vi "运维调试界面.vi"() -> ()   [LabVIEW 2016, in "质控单元V2.lvlib"]
uses:
  <vilib>/Utility/miscctls.llb/LVPointTypeDef.ctl
panel:
  in  "周期设置":bool
  in  "集成干预测试":bool
  in  "平行样测试":bool
  in  "水样测试":bool
  in  "数值":u8
  in  "向前寻道按钮":bool
  in  "向后寻道按钮":bool
  out "质控状态 4":T1
  out "质控状态 3":T1
  out "质控状态 2":T1
  out "质控状态":T1
  out "权限等级":string
  in  "布尔":bool
  out "模块版本号":string
  in  "停止":bool
  in  "参数设置":bool
  in  "连接设置":bool
  in  "调试界面":bool
  in  "加标回收":bool
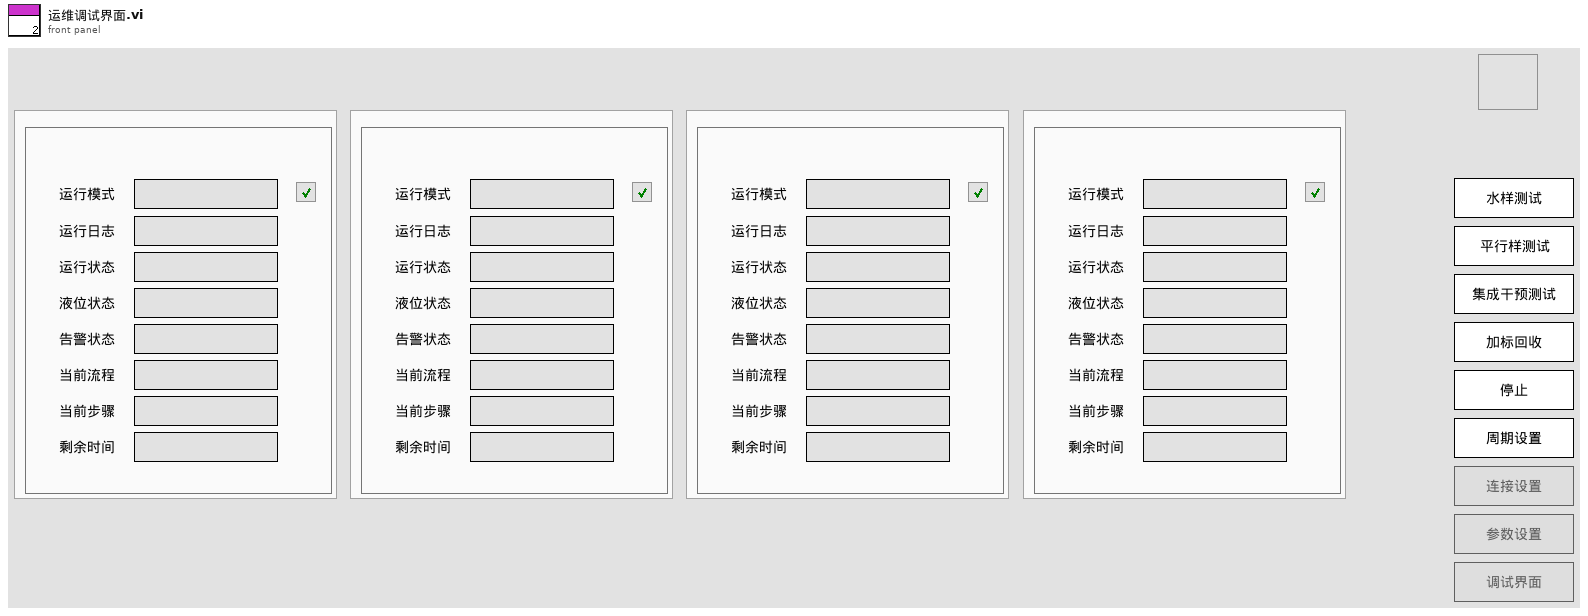
[diagram p1: front panel]
types:
  T1 = typedef "质控单元V2.lvlib/质控状态.ctl" = cluster{"模块名称":string, "通讯状态":bool, "运行模式":string, "运行日志":string, "运行状态":string, "液位状态":string, "告警状态":string, "当前流程":string, "当前步骤":string, "剩余时间":string}
  T2 = typedef "质控单元V2.lvlib/数据流类型.ctl" = cluster{"cmd":enum16{"start", "stop"}, "data":variant}
  T3 = typedef "LVPointTypeDef.ctl" = cluster{"Horizontal":i16, "Vertical":i16}
  T4 = typedef "质控单元V2.lvlib/质控仪器状态显示.ctl" = cluster{"运行模式":string, "运行状态":string, "液位状态":string, "告警状态":string, "当前流程":string, "当前步骤":string, "剩余时间":string}
  T5 = cluster{"氨氮":bool, "总磷":bool, "总氮":bool, "CODMn":bool, "CODCr":bool, "氨氮总磷":bool, "总磷总氮":bool}
  T6 = typedef "质控单元V2.lvlib/质控slave id.ctl" = enum16{"null", "氨氮", "总磷", "总氮", "CODMn", "CODCr"}
  T7 = typedef "质控单元V2.lvlib/测试流程.ctl" = enum16{"加标回收（启动采配水）", "加标回收（不启动采配水）", "水样测试（启动采配水）", "水样测试（不启动采配水）", "平行样测试（启动采配水）", "平行样测试（不启动采配水）", "集成干预测试"}
  T8 = cluster{"启用参数选择":cluster{"氨氮启用":bool, "总磷启用":bool, "总氮启用":bool, "CODMn启用":bool, "CODCr启用":bool}, "流程":T7}
  T9 = cluster{"氨氮启用":bool, "总磷启用":bool, "总氮启用":bool, "CODMn启用":bool, "CODCr启用":bool}
  T10 = enum8{"Enabled", "Disabled", "Disabled and Grayed Out"}
  T11 = cluster{"Major":u16, "Minor":u16, "Fix":u16, "Build":u16}
  T12 = cluster{"氨氮":bool, "总磷":bool, "总氮":bool, "CODMn":bool, "CODCr":bool}
  T13 = cluster{"氨氮":bool, "总磷":bool, "总氮":bool, "CODMn":bool, "CODCr":bool, bool, bool}
  T14 = typedef "ZKTimingControl.lvlib/TimingControl.lvclass/国标控制命令.ctl" = enum16{"加标回收（启动采配水）", "加标回收（不启动采配水）", "水样测试（启动采配水）", "水样测试（不启动采配水）", "平行样测试（启动采配水）", "平行样测试（不启动采配水）", "集成干预测试"}
  T15 = typedef "ZKTimingControl.lvlib/TimingControl.lvclass/测量参数.ctl" = cluster{"氨氮":bool, "总磷":bool, "总氮":bool, "CODMn":bool, "CODCr":bool, "氟化物":bool, "挥发酚":bool}
  T16 = enum32{"Bad", "Idle", "Run top level", "Running"}
  T17 = cluster{"启动参数":cluster{"氨氮启用":bool, "总磷启用":bool, "总氮启用":bool, "CODMn启用":bool, "CODCr启用":bool}, "流程参数":T7}
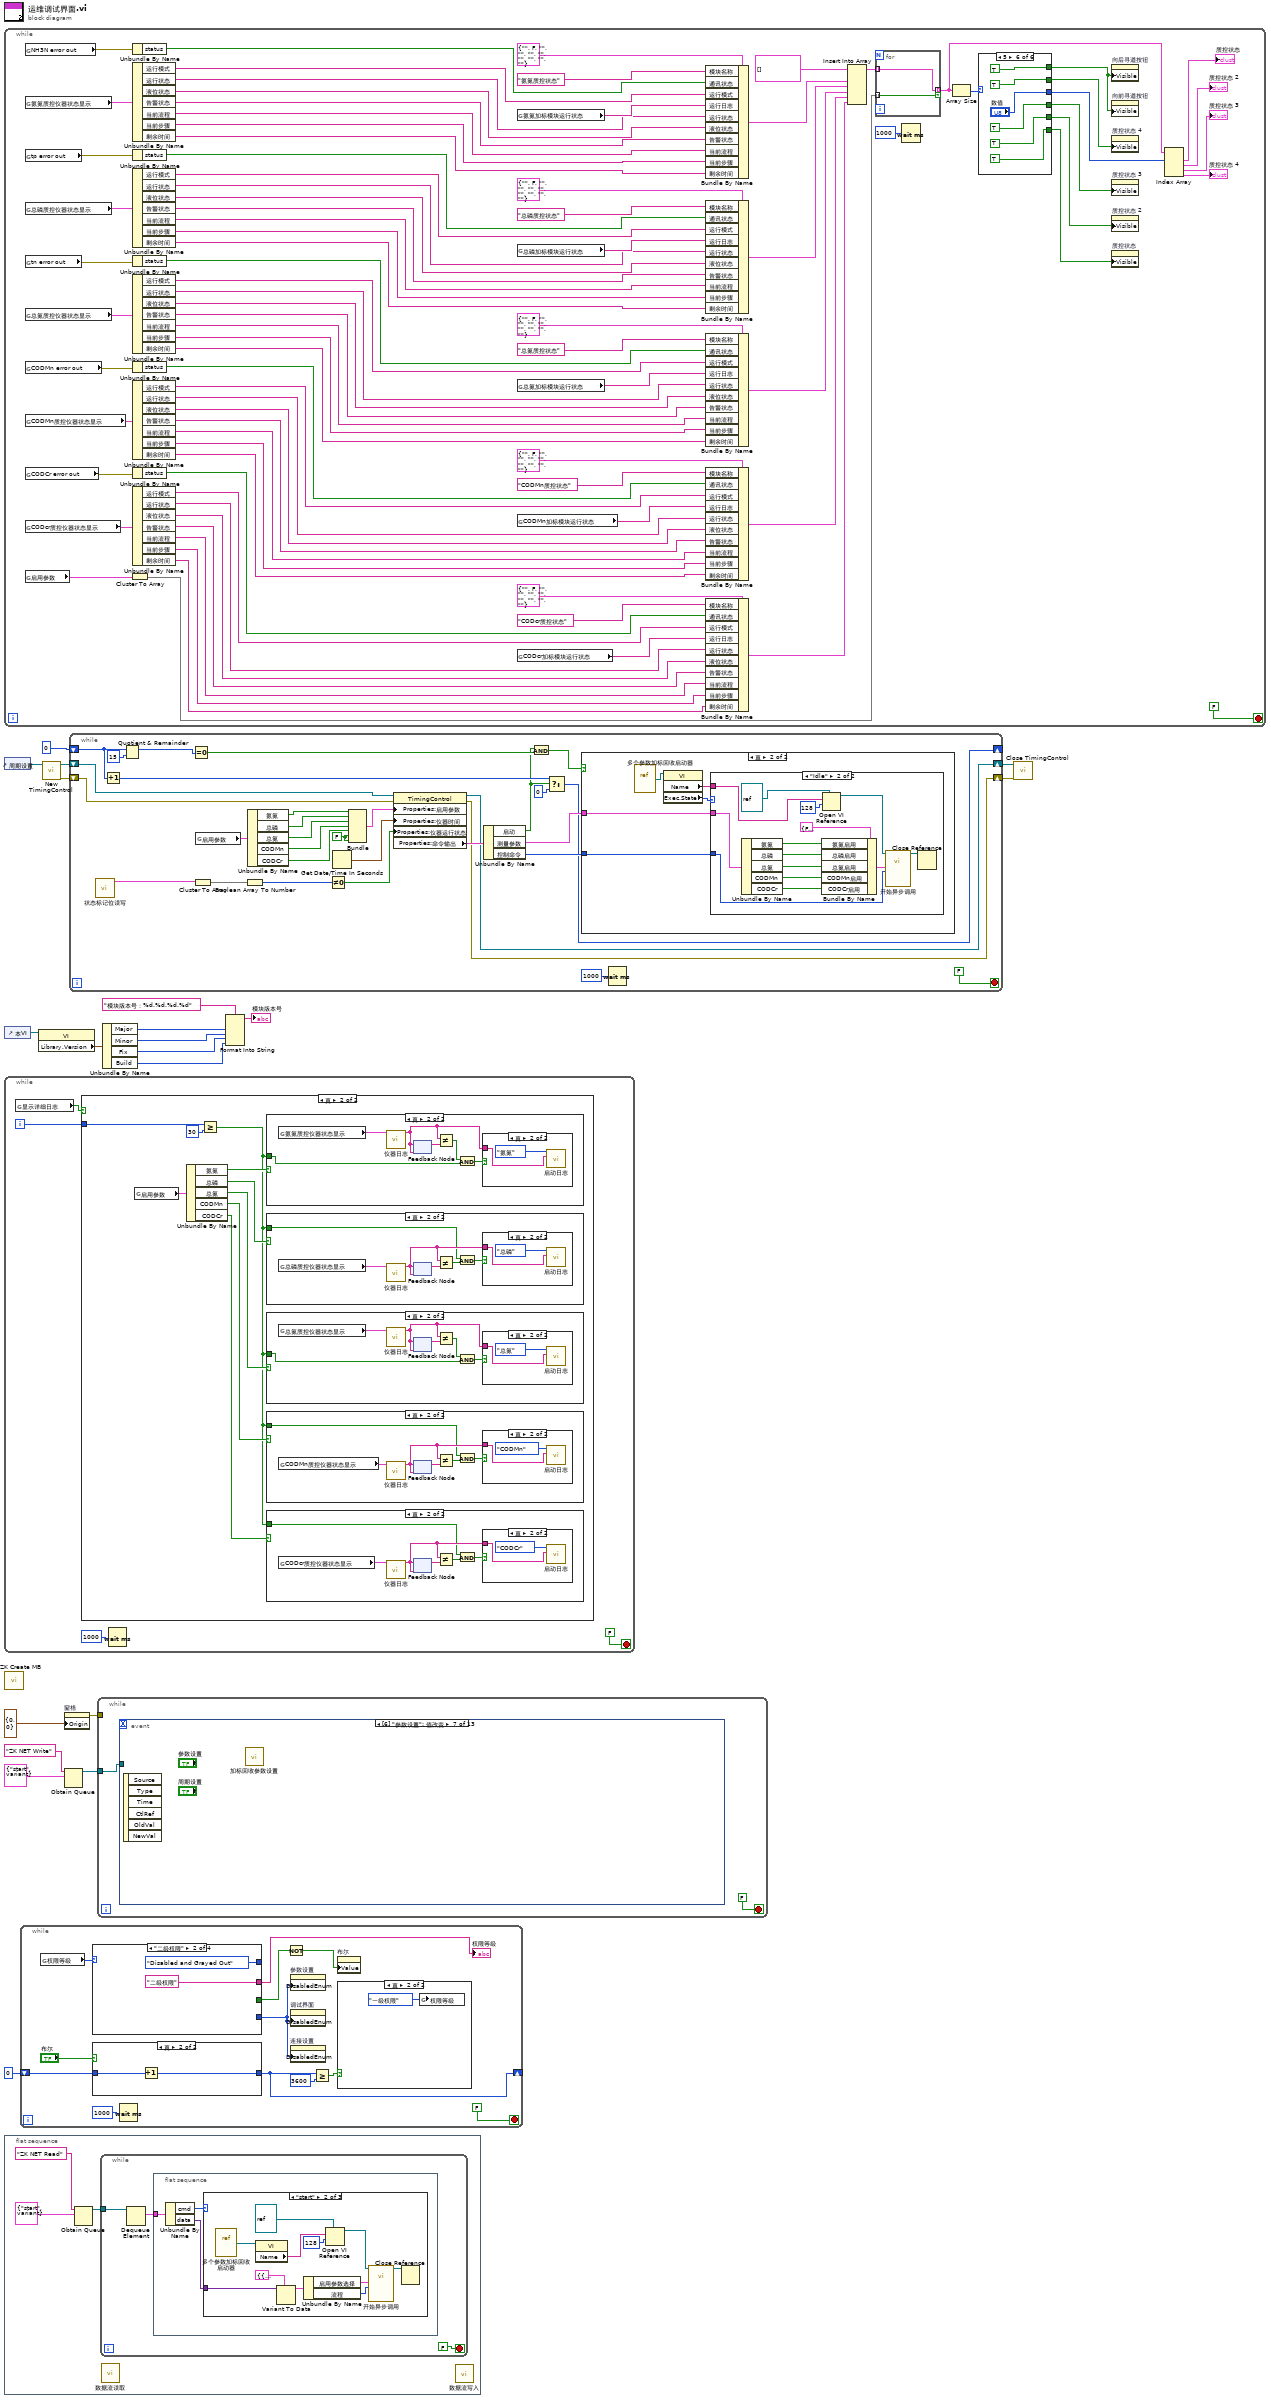
[diagram p0: block diagram]
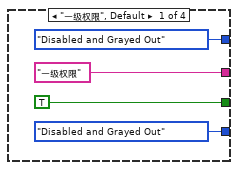
[diagram p13: hidden frame]
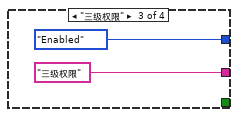
[diagram p14: hidden frame]
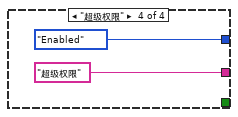
[diagram p15: hidden frame]
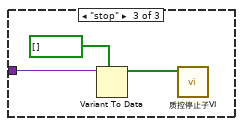
[diagram p19: hidden frame]
diagram:
  n1 = while {
    stop <- FALSE stop-if-true
    n2 = global read "ZK非断电保存全局变量.vi" "NH3N error out"() -> (w105:errorcluster)
    n3 = global read "ZK非断电保存全局变量.vi" "氨氮质控仪器状态显示"() -> (w104:T4)
    n4 = global read "ZK非断电保存全局变量.vi" "tp error out"() -> (w100:errorcluster)
    n5 = global read "ZK非断电保存全局变量.vi" "总磷质控仪器状态显示"() -> (w103:T4)
    n6 = global read "ZK非断电保存全局变量.vi" "tn error out"() -> (w99:errorcluster)
    n7 = global read "ZK非断电保存全局变量.vi" "总氮质控仪器状态显示"() -> (w102:T4)
    n8 = global read "ZK非断电保存全局变量.vi" "CODMn error out"() -> (w106:errorcluster)
    n9 = global read "ZK非断电保存全局变量.vi" "CODMn质控仪器状态显示"() -> (w101:T4)
    n10 = global read "ZK非断电保存全局变量.vi" "CODCr error out"() -> (w37:errorcluster)
    n11 = global read "ZK非断电保存全局变量.vi" "CODcr质控仪器状态显示"() -> (w38:T4)
    n12 = global read "ZK断电保存全局变量.vi" "启用参数"() -> (w34:T5)
    n13 = Cluster To Array(cluster=w34) -> (array=w33:bool[])
    n14 = Unbundle By Name(w105) -> ("status"=w97:bool)
    n15 = Unbundle By Name(w104) -> ("运行模式"=w95:string, "运行状态"=w93:string, "液位状态"=w92:string, "告警状态"=w91:string, "当前流程"=w90:string, "当前步骤"=w89:string, "剩余时间"=w88:string)
    n16 = Unbundle By Name(w100) -> ("status"=w77:bool)
    n17 = Unbundle By Name(w103) -> ("运行模式"=w85:string, "运行状态"=w84:string, "液位状态"=w83:string, "告警状态"=w82:string, "当前流程"=w81:string, "当前步骤"=w80:string, "剩余时间"=w79:string)
    n18 = Unbundle By Name(w99) -> ("status"=w61:bool)
    n19 = Unbundle By Name(w102) -> ("运行模式"=w63:string, "运行状态"=w60:string, "液位状态"=w59:string, "告警状态"=w58:string, "当前流程"=w57:string, "当前步骤"=w56:string, "剩余时间"=w55:string)
    n20 = Unbundle By Name(w106) -> ("status"=w74:bool)
    n21 = Unbundle By Name(w101) -> ("运行模式"=w72:string, "运行状态"=w71:string, "液位状态"=w70:string, "告警状态"=w69:string, "当前流程"=w68:string, "当前步骤"=w67:string, "剩余时间"=w66:string)
    n22 = Unbundle By Name(w37) -> ("status"=w41:bool)
    n23 = Unbundle By Name(w38) -> ("运行模式"=w43:string, "运行状态"=w44:string, "液位状态"=w45:string, "告警状态"=w46:string, "当前流程"=w47:string, "当前步骤"=w48:string, "剩余时间"=w49:string)
    n24 = global read "ZK非断电保存全局变量.vi" "氨氮加标模块运行状态"() -> (w94:string)
    n25 = global read "ZK非断电保存全局变量.vi" "总磷加标模块运行状态"() -> (w86:string)
    n26 = global read "ZK非断电保存全局变量.vi" "总氮加标模块运行状态"() -> (w62:string)
    n27 = global read "ZK非断电保存全局变量.vi" "CODMn加标模块运行状态"() -> (w73:string)
    n28 = global read "ZK非断电保存全局变量.vi" "CODcr加标模块运行状态"() -> (w42:string)
    n29 = Bundle By Name(cluster=T1 {"模块名称"="", "通讯状态"=FALSE, "运行模式"="", "运行日志"="", "运行状态"="", "液位状态"="", "告警状态"="", "当前流程"="", "当前步骤"="", "剩余时间"=""} ("质控状态"), "模块名称"="氨氮质控状态", "通讯状态"=w97, "运行模式"=w95, "运行日志"=w94, "运行状态"=w93, "液位状态"=w92, "告警状态"=w91, "当前流程"=w90, "当前步骤"=w89, "剩余时间"=w88) -> (w54:T1)
    n30 = Bundle By Name(cluster=T1 {"模块名称"="", "通讯状态"=FALSE, "运行模式"="", "运行日志"="", "运行状态"="", "液位状态"="", "告警状态"="", "当前流程"="", "当前步骤"="", "剩余时间"=""} ("质控状态"), "模块名称"="总磷质控状态", "通讯状态"=w77, "运行模式"=w85, "运行日志"=w86, "运行状态"=w84, "液位状态"=w83, "告警状态"=w82, "当前流程"=w81, "当前步骤"=w80, "剩余时间"=w79) -> (w52:T1)
    n31 = Bundle By Name(cluster=T1 {"模块名称"="", "通讯状态"=FALSE, "运行模式"="", "运行日志"="", "运行状态"="", "液位状态"="", "告警状态"="", "当前流程"="", "当前步骤"="", "剩余时间"=""} ("质控状态"), "模块名称"="总氮质控状态", "通讯状态"=w61, "运行模式"=w63, "运行日志"=w62, "运行状态"=w60, "液位状态"=w59, "告警状态"=w58, "当前流程"=w57, "当前步骤"=w56, "剩余时间"=w55) -> (w51:T1)
    n32 = Bundle By Name(cluster=T1 {"模块名称"="", "通讯状态"=FALSE, "运行模式"="", "运行日志"="", "运行状态"="", "液位状态"="", "告警状态"="", "当前流程"="", "当前步骤"="", "剩余时间"=""} ("质控状态"), "模块名称"="CODMn质控状态", "通讯状态"=w74, "运行模式"=w72, "运行日志"=w73, "运行状态"=w71, "液位状态"=w70, "告警状态"=w69, "当前流程"=w68, "当前步骤"=w67, "剩余时间"=w66) -> (w50:T1)
    n33 = Bundle By Name(cluster=T1 {"模块名称"="", "通讯状态"=FALSE, "运行模式"="", "运行日志"="", "运行状态"="", "液位状态"="", "告警状态"="", "当前流程"="", "当前步骤"="", "剩余时间"=""} ("质控状态"), "模块名称"="CODcr质控状态", "通讯状态"=w41, "运行模式"=w43, "运行日志"=w42, "运行状态"=w44, "液位状态"=w45, "告警状态"=w46, "当前流程"=w47, "当前步骤"=w48, "剩余时间"=w49) -> (w36:T1)
    n34 = Insert Into Array(array=T1[] [] ("数组"), new element #1=w54, new element #2=w52, new element #3=w51, new element #4=w50, new element #5=w36) -> (w35:T1[])  [unwired: 1 in]
    n35 = for {
      tunnel: w35 -> [w130] mode=indexing
      tunnel: w33 -> [w129] mode=indexing
      tunnel: [w130] -> w28 mode=indexing if=w129
    }
    n36 = Wait (ms)(milliseconds to wait=u32 1000 ("等待时间（毫秒）")) -> ()  [unwired: 1 out]
    n37 = Array Size(array=w28) -> (size(s)=w27:i32)
    n38 = case shown="5" w27 {
      tunnel: [FALSE TRUE TRUE TRUE TRUE TRUE] -> w26
      tunnel: [FALSE _ TRUE TRUE TRUE TRUE] -> w25
      tunnel: [FALSE _ _ TRUE TRUE TRUE] -> w24
      tunnel: [FALSE _ _ _ TRUE TRUE] -> w23
      tunnel: [_ _ _ _ _ TRUE] -> w22
      tunnel: [_ _ _ _ _ "数值"] -> w21
      frame 0, Default {
      }
      frame 1 {
      }
      frame 2 {
      }
      frame 3 {
      }
      frame 4 {
      }
      frame 5 {
      }
    }
    n39 = property on="向后寻道按钮" class="Bool"("Visible"=w22) -> ()  [unwired: 2 in, 2 out]
    n40 = property on="向前寻道按钮" class="Bool"("Visible"=w22) -> ()  [unwired: 2 in, 2 out]
    n41 = property on="质控状态 4" class="Clust (严格)"("Visible"=w23) -> ()  [unwired: 2 in, 2 out]
    n42 = property on="质控状态 3" class="Clust (严格)"("Visible"=w24) -> ()  [unwired: 2 in, 2 out]
    n43 = property on="质控状态 2" class="Clust (严格)"("Visible"=w25) -> ()  [unwired: 2 in, 2 out]
    n44 = property on="质控状态" class="Clust (严格)"("Visible"=w26) -> ()  [unwired: 2 in, 2 out]
    n45 = Index Array(array=w28, index #1=w21) -> (element #1=→"质控状态":T1, element #2=→"质控状态 2":T1, element #3=→"质控状态 3":T1, element #4=→"质控状态 4":T1)  [unwired: 3 in]
  }
  n46 = control-ref of="周期设置"() -> (w1:refnum<vi>)
  n47 = control-ref of="本VI"() -> (w18:refnum<vi>)
  n48 = while {
    i -> [w132]
    stop <- FALSE stop-if-true
    n49 = global read "ZK断电保存全局变量.vi" "显示详细日志"() -> (w131:bool)
    n50 = case shown="真" w131 {
      tunnel: w132 -> [_ w137]
      frame False {
      }
      frame True {
        n51 = global read "ZK断电保存全局变量.vi" "启用参数"() -> (w143:T5)
        n52 = Unbundle By Name(w143) -> ("氨氮"=w142:bool, "总磷"=w141:bool, "总氮"=w140:bool, "CODMn"=w139:bool, "CODCr"=w138:bool)
        n53 = Greater Or Equal?(x=w137, y=30) -> (x >= y?=w135:bool)
        n54 = case shown="真" w142 {
          tunnel: w135 -> [_ w176]
          frame False {
          }
          frame True {
            n55 = global read "ZK非断电保存全局变量.vi" "氨氮质控仪器状态显示"() -> (w181:T4)
            n56 = call "仪器日志.vi"("质控仪器状态显示"=w181) -> ("仪器日志"=w179:string)  [unwired: 10 in]
            n57 = feedback-in #1(w179) -> ()
            n58 = feedback #1(w179) -> (w180:string)
            n59 = Not Equal?(x=w179, y=w180) -> (x != y?=w178:bool)
            n60 = And(x=w178, y=w176) -> (x .and. y?=w177:bool)
            n61 = case shown="真" w177 {
              tunnel: w179 -> [_ w182]
              frame False {
              }
              frame True {
                n62 = call "启动日志.vi"("日志信息"=w182, "Slave ID"=质控slave_id."氨氮") -> ()  [unwired: 9 in, 1 out]
              }
            }
          }
        }
        n63 = case shown="真" w141 {
          tunnel: w135 -> [_ w168]
          frame False {
          }
          frame True {
            n64 = global read "ZK非断电保存全局变量.vi" "总磷质控仪器状态显示"() -> (w170:T4)
            n65 = call "仪器日志.vi"("质控仪器状态显示"=w170) -> ("仪器日志"=w172:string)  [unwired: 10 in]
            n66 = feedback #2(w172) -> (w173:string)
            n67 = feedback-in #2(w172) -> ()
            n68 = Not Equal?(x=w172, y=w173) -> (x != y?=w171:bool)
            n69 = And(x=w168, y=w171) -> (x .and. y?=w169:bool)
            n70 = case shown="真" w169 {
              tunnel: w172 -> [_ w174]
              frame False {
              }
              frame True {
                n71 = call "启动日志.vi"("日志信息"=w174, "Slave ID"=质控slave_id."总磷") -> ()  [unwired: 9 in, 1 out]
              }
            }
          }
        }
        n72 = case shown="真" w140 {
          tunnel: w135 -> [_ w160]
          frame False {
          }
          frame True {
            n73 = global read "ZK非断电保存全局变量.vi" "总氮质控仪器状态显示"() -> (w162:T4)
            n74 = call "仪器日志.vi"("质控仪器状态显示"=w162) -> ("仪器日志"=w164:string)  [unwired: 10 in]
            n75 = feedback #3(w164) -> (w165:string)
            n76 = feedback-in #3(w164) -> ()
            n77 = Not Equal?(x=w164, y=w165) -> (x != y?=w163:bool)
            n78 = And(x=w163, y=w160) -> (x .and. y?=w161:bool)
            n79 = case shown="真" w161 {
              tunnel: w164 -> [_ w166]
              frame False {
              }
              frame True {
                n80 = call "启动日志.vi"("日志信息"=w166, "Slave ID"=质控slave_id."总氮") -> ()  [unwired: 9 in, 1 out]
              }
            }
          }
        }
        n81 = case shown="真" w139 {
          tunnel: w135 -> [_ w152]
          frame False {
          }
          frame True {
            n82 = global read "ZK非断电保存全局变量.vi" "CODMn质控仪器状态显示"() -> (w154:T4)
            n83 = call "仪器日志.vi"("质控仪器状态显示"=w154) -> ("仪器日志"=w156:string)  [unwired: 10 in]
            n84 = feedback #4(w156) -> (w157:string)
            n85 = feedback-in #4(w156) -> ()
            n86 = Not Equal?(x=w156, y=w157) -> (x != y?=w155:bool)
            n87 = And(x=w152, y=w155) -> (x .and. y?=w153:bool)
            n88 = case shown="真" w153 {
              tunnel: w156 -> [_ w158]
              frame False {
              }
              frame True {
                n89 = call "启动日志.vi"("日志信息"=w158, "Slave ID"=质控slave_id."CODMn") -> ()  [unwired: 9 in, 1 out]
              }
            }
          }
        }
        n90 = case shown="真" w138 {
          tunnel: w135 -> [_ w144]
          frame False {
          }
          frame True {
            n91 = global read "ZK非断电保存全局变量.vi" "CODcr质控仪器状态显示"() -> (w146:T4)
            n92 = call "仪器日志.vi"("质控仪器状态显示"=w146) -> ("仪器日志"=w148:string)  [unwired: 10 in]
            n93 = feedback #5(w148) -> (w149:string)
            n94 = feedback-in #5(w148) -> ()
            n95 = Not Equal?(x=w148, y=w149) -> (x != y?=w147:bool)
            n96 = And(x=w144, y=w147) -> (x .and. y?=w145:bool)
            n97 = case shown="真" w145 {
              tunnel: w148 -> [_ w150]
              frame False {
              }
              frame True {
                n98 = call "启动日志.vi"("日志信息"=w150, "Slave ID"=质控slave_id."CODCr") -> ()  [unwired: 9 in, 1 out]
              }
            }
          }
        }
      }
    }
    n99 = Wait (ms)(milliseconds to wait=u32 1000 ("等待时间（毫秒）")) -> ()  [unwired: 1 out]
  }
  n100 = call "ZK Create MB.vi"() -> ()  [unwired: 12 in]
  n101 = flat-sequence {
    frame #0 {
      n102 = Obtain Queue(name (unnamed)="ZK NET Read" ("名称（未命名）"), element data type=T2 {"cmd"=enum."start", "data"=variant} ("簇")) -> (queue out=w185:refnum<queue>)  [unwired: 3 in, 2 out]
      n103 = while {
        tunnel: w185 -> [w189]
        stop <- FALSE stop-if-true
        n104 = Dequeue Element(queue=w189) -> (element=w187:T2)  [unwired: 2 in, 3 out]
        n105 = flat-sequence {
          tunnel: w187 -> [w192]
          frame #0 {
            n106 = Unbundle By Name(w192) -> ("cmd"=w191:enum16{"start", "stop"}, "data"=w190:variant)
            n107 = case shown="\"start\"" w191 {
              tunnel: w190 -> [_ w198 w206]
              frame Default {
              }
              frame "start" {
                n108 = vi-ref "多个参数加标回收启动器.vi"() -> (w203:refnum<vi>)
                n109 = property class="VI"(reference=w203) -> ("Name"=w202:string)  [unwired: 1 in, 2 out]
                n110 = Variant To Data(type=T8 {"启用参数选择"={"氨氮启用"=FALSE, "总磷启用"=FALSE, "总氮启用"=FALSE, "CODMn启用"=FALSE, "CODCr启用"=FALSE}, "流程"=enum."加标回收（启动采配水）"} ("data"), Variant=w198) -> (data=w196:T8)  [unwired: 1 in, 1 out]
                n111 = Unbundle By Name(w196) -> ("启用参数选择"=w195:T9, "流程"=w194:T7)
                n112 = Open VI Reference(type specifier VI Refnum (for type only)=refnum<vi> refnum, vi path=w202, options=128 ("选项")) -> (vi reference=w200:refnum<vi>)  [unwired: 3 in, 1 out]
                n113 = call-by-ref "开始异步调用"(reference=w200, "流程"=w194, "启用参数选择"=w195) -> (reference out=w199:refnum<vi>)  [unwired: 11 in, 1 out]
                n114 = Close Reference(reference=w199) -> ()  [unwired: 1 in, 1 out]
              }
              frame "stop" {
                n115 = Variant To Data(type=bool[] [] ("数组"), Variant=w206) -> (data=w204:bool[])  [unwired: 1 in, 1 out]
                n116 = call "质控停止子VI.vi"("数组"=w204) -> ()  [unwired: 11 in]
              }
            }
          }
        }
      }
      n117 = call "数据流读取.vi"() -> ()  [unwired: 12 in]
      n118 = call "数据流写入.vi"() -> ()  [unwired: 12 in]
    }
  }
  n119 = while {
    shift-right: [w217] -> _
    shift-left: 0 -> [w218]
    stop <- FALSE stop-if-true
    n120 = global read "ZK非断电保存全局变量.vi" "权限等级"() -> (w212:enum16{"一级权限", "二级权限", "三级权限", "超级权限"})
    n121 = case shown="\"二级权限\"" w212 {
      tunnel: [T10."Disabled and Grayed Out" ("禁用") _ _ _] -> w207
      tunnel: ["一级权限" "二级权限" "三级权限" "超级权限"] -> w210
      tunnel: [TRUE ("布尔") _ _ _] -> w209
      tunnel: [T10."Disabled and Grayed Out" ("禁用") T10."Disabled and Grayed Out" ("禁用") T10."Enabled" ("禁用") T10."Enabled" ("禁用")] -> _
      frame "一级权限", Default {
      }
      frame "二级权限" {
      }
      frame "三级权限" {
      }
      frame "超级权限" {
      }
    }
    "权限等级" <- w210
    n122 = case shown="真" "布尔" {
      tunnel: w218 -> [_ w231]
      tunnel: [_ w230] -> w217
      frame False {
      }
      frame True {
        n123 = Increment(x=w231) -> (x+1=w230:i32)
      }
    }
    n124 = Wait (ms)(milliseconds to wait=u32 1000 ("等待时间（毫秒）")) -> ()  [unwired: 1 out]
    n125 = Not(x=w209) -> (.not. x?=w208:bool)
    n126 = property on="参数设置" class="Bool"("DisabledEnum"=w207) -> ()  [unwired: 2 in, 2 out]
    n127 = property on="调试界面" class="Bool"("DisabledEnum"=w207) -> ()  [unwired: 2 in, 2 out]
    n128 = property on="连接设置" class="Bool"("DisabledEnum"=w207) -> ()  [unwired: 2 in, 2 out]
    n129 = Greater Or Equal?(x=w217, y=3600) -> (x >= y?=w215:bool)
    n130 = property on="布尔" class="Bool (严格)"("Value"=w208) -> ()  [unwired: 2 in, 2 out]
    n131 = case shown="真" w215 {
      frame False {
      }
      frame True {
        n132 = global write "ZK非断电保存全局变量.vi" "权限等级"(enum16{"一级权限", "二级权限", "三级权限", "超级权限"}."一级权限" ("权限等级")) -> ()
      }
    }
  }
  n133 = property class="VI"(reference=w18) -> ("Library.Version"=w17:T11)  [unwired: 1 in, 2 out]
  n134 = call "New TimingControl.vi"("Reference"=w1) -> ("error out"=w4:errorcluster, "TimingControl out"=w5:refnum<class "TimingControl.lvclass">)  [unwired: 9 in]
  n135 = property on="窗格" class="Pane"("Origin"=T3 {"Horizontal"=0, "Vertical"=0} ("原点")) -> (error out=w19:errorcluster)  [unwired: 2 in, 1 out]
  n136 = Obtain Queue(name (unnamed)="ZK NET Write" ("名称（未命名）"), element data type=T2 {"cmd"=enum."start", "data"=variant} ("簇")) -> (queue out=w9:refnum<queue>)  [unwired: 3 in, 2 out]
  n137 = while {
    shift-right: [w248] -> _
    shift-left: 0 -> [w247]
    shift-right: [w235] -> w3
    shift-left: w5 -> [w241]
    shift-right: [w234] -> w2
    shift-left: w4 -> [w240]
    stop <- FALSE stop-if-true
    w232 = FALSE
    n138 = call "状态标记位读写.vi"() -> ("运维标记位"=w233:T12)  [unwired: 11 in]
    n139 = Increment(x=w247) -> (x+1=w250:i32)
    n140 = Quotient & Remainder(x=w247, y=15) -> (x-y*floor(x/y)=w245:i32)  [unwired: 1 out]
    n141 = Equal To 0?(x=w245) -> (x = 0?=w244:bool)
    n142 = Cluster To Array(cluster=w233) -> (array=w258:bool[])
    n143 = global read "ZK断电保存全局变量.vi" "启用参数"() -> (w256:T5)
    n144 = Boolean Array To Number(Boolean array=w258) -> (number=w257:u32)
    n145 = Unbundle By Name(w256) -> ("氨氮"=w255:bool, "总磷"=w254:bool, "总氮"=w253:bool, "CODMn"=w252:bool, "CODCr"=w251:bool)
    n146 = Not Equal To 0?(x=w257) -> (x != 0?=w238:bool)
    n147 = Get Date/Time In Seconds() -> (seconds since 1Jan1904=w239:timestamp)
    n148 = Bundle("氨氮"=w255, "总磷"=w254, "总氮"=w253, "CODMn"=w252, "CODCr"=w251, w232, w232) -> (w237:T13)  [unwired: 1 in]
    n149 = property class="TimingControl"(reference=w241, error in=w240, "Properties:启用参数"=w237, "Properties:仪器时间"=w239, "Properties:仪器运行状态"=w238) -> (reference out=w235:refnum<class "TimingControl.lvclass">, error out=w234:errorcluster, "Properties:命令输出"=w236:cluster{"启动":bool, "控制命令":T14, "测量参数":T15})
    n150 = Unbundle By Name(w236) -> ("启动"=w243:bool, "测量参数"=w260:T15, "控制命令"=w259:T14)
    n151 = And(x=w243, y=w244) -> (x .and. y?=w242:bool)
    n152 = Select(t=w250, s=w243, f=0) -> (s? t:f=w248:i32)
    n153 = case shown="真" w242 {
      tunnel: w260 -> [_ w265]
      tunnel: w259 -> [_ w264]
      frame False {
      }
      frame True {
        n154 = vi-ref "多个参数加标回收启动器.vi"() -> (w266:refnum<vi>)
        n155 = property class="VI"(reference=w266) -> ("Name"=w267:string, "Exec.State"=w263:T16)  [unwired: 1 in, 2 out]
        n156 = case shown="\"Idle\"" w263 {
          tunnel: w267 -> [_ w278]
          tunnel: w265 -> [_ w273]
          tunnel: w264 -> [_ w277]
          frame "Bad", Default {
          }
          frame "Idle" {
            n157 = Unbundle By Name(w273) -> ("氨氮"=w272:bool, "总磷"=w271:bool, "总氮"=w270:bool, "CODMn"=w269:bool, "CODCr"=w268:bool)
            n158 = Bundle By Name(cluster=T9 {"氨氮启用"=FALSE, "总磷启用"=FALSE, "总氮启用"=FALSE, "CODMn启用"=FALSE, "CODCr启用"=FALSE} ("启用参数选择"), "氨氮启用"=w272, "总磷启用"=w271, "总氮启用"=w270, "CODMn启用"=w269, "CODCr启用"=w268) -> (w274:T9)
            n159 = Open VI Reference(type specifier VI Refnum (for type only)=refnum<vi> refnum, vi path=w278, options=128 ("选项")) -> (vi reference=w280:refnum<vi>)  [unwired: 3 in, 1 out]
            n160 = call-by-ref "开始异步调用"(reference=w280, "流程"=w277, "启用参数选择"=w274) -> (reference out=w281:refnum<vi>)  [unwired: 11 in, 1 out]
            n161 = Close Reference(reference=w281) -> ()  [unwired: 1 in, 1 out]
          }
        }
      }
    }
    n162 = Wait (ms)(milliseconds to wait=u32 1000 ("等待时间（毫秒）")) -> ()  [unwired: 1 out]
  }
  n163 = while {
    tunnel: w19 -> [_]
    tunnel: w9 -> [w282]
    stop <- FALSE stop-if-true
    n164 = event shown="[6] \"参数设置\": 值改变" {
      selector: _ -> [_ _ _ _ _ _ _ _ _ _ _ _ _]
      dyn-events: _ -> [_ _ _ _ _ _ _ _ _ _ _ _ _]
      timeout: _ -> [_ _ _ _ _ _ _ _ _ _ _ _ _]
      tunnel: w282 -> [_ _ _ _ _ _ _ w295 w313 w331 w349 w369 _]
      event Timeout {
        n165 = event-data() -> ()  [unwired: 1 in, 3 out]
      }
      event "布尔": Value Change {
        n166 = event-data() -> ("NewVal"=w284:bool)  [unwired: 1 in, 3 out]
        n167 = case shown="真" w284 {
          frame False {
            n168 = global write "ZK非断电保存全局变量.vi" "权限等级"(enum16{"一级权限", "二级权限", "三级权限", "超级权限"}."一级权限" ("权限等级")) -> ()
          }
          frame True {
            n169 = global read "ZK非断电保存全局变量.vi" "权限密码"() -> (w288:u32[])
            n170 = global read "ZK非断电保存全局变量.vi" "权限等级"() -> (w286:enum16{"一级权限", "二级权限", "三级权限", "超级权限"})
            n171 = call "密码权限设置.vi"("权限输入"=w286, "权限密码"=w288) -> ("权限输出"=w287:enum16{"一级权限", "二级权限", "三级权限", "超级权限"})  [unwired: 9 in]
            n172 = global write "ZK非断电保存全局变量.vi" "权限等级"(w287) -> ()
          }
        }
      }
      event "权限等级": Mouse Down {
        n173 = event-data() -> ()  [unwired: 1 in, 8 out]
        n174 = global read "ZK非断电保存全局变量.vi" "权限密码"() -> (w291:u32[])
        n175 = global read "ZK非断电保存全局变量.vi" "权限等级"() -> (w289:enum16{"一级权限", "二级权限", "三级权限", "超级权限"})
        n176 = call "密码权限设置.vi"("权限输入"=w289, "权限密码"=w291) -> ("权限输出"=w290:enum16{"一级权限", "二级权限", "三级权限", "超级权限"})  [unwired: 9 in]
        n177 = global write "ZK非断电保存全局变量.vi" "权限等级"(w290) -> ()
      }
      event "调试界面": Value Change {
        n178 = event-data() -> ()  [unwired: 1 in, 6 out]
        n179 = call "加标回收调试界面.vi"() -> ()  [unwired: 12 in]
      }
      event "向后寻道按钮": Value Change {
        n180 = event-data() -> ()  [unwired: 1 in, 6 out]
        n181 = property on="数值" class="DigNum (严格)"("Value"=u8 1 ("数值")) -> ()  [unwired: 2 in, 2 out]
      }
      event "向前寻道按钮": Value Change {
        n182 = event-data() -> ()  [unwired: 1 in, 6 out]
        n183 = property on="数值" class="DigNum (严格)"("Value"=u8 0 ("数值")) -> ()  [unwired: 2 in, 2 out]
      }
      event "参数设置": Value Change {
        n184 = event-data() -> ()  [unwired: 1 in, 6 out]
        n185 = call "加标回收参数设置.vi"() -> ()  [unwired: 12 in]
      }
      event "加标回收": Value Change {
        n186 = event-data() -> ()  [unwired: 1 in, 6 out]
        n187 = call "加标回收启动对话框.vi"("测试模式"=enum16{"水样测试", "平行样测试", "加标回收", "集成干预测试"}."加标回收") -> ("流程参数"=w296:T7, "启动参数"=w297:T9, "check ？"=w298:bool)  [unwired: 8 in]
        n188 = case shown="真" w298 {
          tunnel: w297 -> [_ w305]
          tunnel: w296 -> [_ w304]
          tunnel: w295 -> [_ w306]
          frame False {
          }
          frame True {
            n189 = Bundle("启动参数"=w305, "流程参数"=w304) -> (w301:T17)  [unwired: 1 in]
            n190 = vi-ref "多个参数加标回收启动器.vi"() -> (w311:refnum<vi>)
            n191 = property class="VI"(reference=w311) -> ("Name"=w310:string)  [unwired: 1 in, 2 out]
            n192 = Bundle By Name(cluster=T2 {"cmd"=enum."start", "data"=variant} ("簇"), "cmd"=enum16{"start", "stop"}."start", "data"=w301) -> (w300:T2)
            n193 = Enqueue Element(queue=w306, element=w300) -> ()  [unwired: 2 in, 3 out]
            n194 = Open VI Reference(type specifier VI Refnum (for type only)=refnum<vi> refnum, vi path=w310, options=128 ("选项")) -> (vi reference=w308:refnum<vi>)  [unwired: 3 in, 1 out]
            n195 = call-by-ref "开始异步调用"(reference=w308, "流程"=w304, "启用参数选择"=w305) -> (reference out=w307:refnum<vi>)  [unwired: 11 in, 1 out]
            n196 = Close Reference(reference=w307) -> ()  [unwired: 1 in, 1 out]
          }
        }
      }
      event "水样测试": Value Change {
        n197 = event-data() -> ()  [unwired: 1 in, 6 out]
        n198 = call "加标回收启动对话框.vi"("测试模式"=enum16{"水样测试", "平行样测试", "加标回收", "集成干预测试"}."水样测试") -> ("流程参数"=w314:T7, "启动参数"=w315:T9, "check ？"=w316:bool)  [unwired: 8 in]
        n199 = case shown="真" w316 {
          tunnel: w315 -> [_ w323]
          tunnel: w314 -> [_ w322]
          tunnel: w313 -> [_ w324]
          frame False {
          }
          frame True {
            n200 = Bundle("启动参数"=w323, "流程参数"=w322) -> (w319:T17)  [unwired: 1 in]
            n201 = vi-ref "多个参数加标回收启动器.vi"() -> (w329:refnum<vi>)
            n202 = property class="VI"(reference=w329) -> ("Name"=w328:string)  [unwired: 1 in, 2 out]
            n203 = Bundle By Name(cluster=T2 {"cmd"=enum."start", "data"=variant} ("簇"), "cmd"=enum16{"start", "stop"}."start", "data"=w319) -> (w318:T2)
            n204 = Enqueue Element(queue=w324, element=w318) -> ()  [unwired: 2 in, 3 out]
            n205 = Open VI Reference(type specifier VI Refnum (for type only)=refnum<vi> refnum, vi path=w328, options=128 ("选项")) -> (vi reference=w326:refnum<vi>)  [unwired: 3 in, 1 out]
            n206 = call-by-ref "开始异步调用"(reference=w326, "流程"=w322, "启用参数选择"=w323) -> (reference out=w325:refnum<vi>)  [unwired: 11 in, 1 out]
            n207 = Close Reference(reference=w325) -> ()  [unwired: 1 in, 1 out]
          }
        }
      }
      event "平行样测试": Value Change {
        n208 = event-data() -> ()  [unwired: 1 in, 6 out]
        n209 = call "加标回收启动对话框.vi"("测试模式"=enum16{"水样测试", "平行样测试", "加标回收", "集成干预测试"}."平行样测试") -> ("流程参数"=w332:T7, "启动参数"=w333:T9, "check ？"=w334:bool)  [unwired: 8 in]
        n210 = case shown="真" w334 {
          tunnel: w333 -> [_ w341]
          tunnel: w332 -> [_ w340]
          tunnel: w331 -> [_ w342]
          frame False {
          }
          frame True {
            n211 = Bundle("启动参数"=w341, "流程参数"=w340) -> (w337:T17)  [unwired: 1 in]
            n212 = vi-ref "多个参数加标回收启动器.vi"() -> (w347:refnum<vi>)
            n213 = property class="VI"(reference=w347) -> ("Name"=w346:string)  [unwired: 1 in, 2 out]
            n214 = Bundle By Name(cluster=T2 {"cmd"=enum."start", "data"=variant} ("簇"), "cmd"=enum16{"start", "stop"}."start", "data"=w337) -> (w336:T2)
            n215 = Enqueue Element(queue=w342, element=w336) -> ()  [unwired: 2 in, 3 out]
            n216 = Open VI Reference(type specifier VI Refnum (for type only)=refnum<vi> refnum, vi path=w346, options=128 ("选项")) -> (vi reference=w344:refnum<vi>)  [unwired: 3 in, 1 out]
            n217 = call-by-ref "开始异步调用"(reference=w344, "流程"=w340, "启用参数选择"=w341) -> (reference out=w343:refnum<vi>)  [unwired: 11 in, 1 out]
            n218 = Close Reference(reference=w343) -> ()  [unwired: 1 in, 1 out]
          }
        }
      }
      event "集成干预测试": Value Change {
        n219 = event-data() -> ()  [unwired: 1 in, 6 out]
        n220 = call "加标回收启动对话框.vi"("测试模式"=enum16{"水样测试", "平行样测试", "加标回收", "集成干预测试"}."集成干预测试") -> ("流程参数"=w350:T7, "启动参数"=w351:T9, "check ？"=w352:bool)  [unwired: 8 in]
        n221 = case shown="真" w352 {
          tunnel: w351 -> [_ w359]
          tunnel: w350 -> [_ w358]
          tunnel: w349 -> [_ w360]
          frame False {
          }
          frame True {
            n222 = Bundle("启动参数"=w359, "流程参数"=w358) -> (w355:T17)  [unwired: 1 in]
            n223 = vi-ref "多个参数加标回收启动器.vi"() -> (w365:refnum<vi>)
            n224 = property class="VI"(reference=w365) -> ("Name"=w364:string)  [unwired: 1 in, 2 out]
            n225 = Bundle By Name(cluster=T2 {"cmd"=enum."start", "data"=variant} ("簇"), "cmd"=enum16{"start", "stop"}."start", "data"=w355) -> (w354:T2)
            n226 = Enqueue Element(queue=w360, element=w354) -> ()  [unwired: 2 in, 3 out]
            n227 = Open VI Reference(type specifier VI Refnum (for type only)=refnum<vi> refnum, vi path=w364, options=128 ("选项")) -> (vi reference=w362:refnum<vi>)  [unwired: 3 in, 1 out]
            n228 = call-by-ref "开始异步调用"(reference=w362, "流程"=w358, "启用参数选择"=w359) -> (reference out=w361:refnum<vi>)  [unwired: 11 in, 1 out]
            n229 = Close Reference(reference=w361) -> ()  [unwired: 1 in, 1 out]
          }
        }
      }
      event "停止": Value Change {
        n230 = event-data() -> ()  [unwired: 1 in, 6 out]
        n231 = Flush Queue(queue=w369) -> (queue out=w368:refnum<queue>)  [unwired: 1 in, 2 out]
        n232 = call "加标回收停止对话框.vi"() -> ("数组"=w367:bool[], "check？"=w366:bool)  [unwired: 10 in]
        n233 = case shown="真" w366 {
          tunnel: w368 -> [_ w374]
          tunnel: w367 -> [_ w370]
          frame False {
          }
          frame True {
            n234 = call "质控停止子VI.vi"("数组"=w370) -> ()  [unwired: 11 in]
            n235 = Bundle By Name(cluster=T2 {"cmd"=enum."start", "data"=variant} ("簇"), "cmd"=enum16{"start", "stop"}."stop", "data"=w370) -> (w371:T2)
            n236 = Enqueue Element(queue=w374, element=w371) -> ()  [unwired: 2 in, 3 out]
          }
        }
      }
      event "连接设置": Value Change {
        n237 = event-data() -> ()  [unwired: 1 in, 6 out]
        n238 = call "串口配置.vi"() -> ()  [unwired: 12 in]
      }
    }
  }
  n239 = Unbundle By Name(w17) -> ("Major"=w15:u16, "Minor"=w14:u16, "Fix"=w13:u16, "Build"=w12:u16)
  n240 = Format Into String(format string="模块版本号：%d.%d.%d.%d" ("格式字符串"), w15, w14, w13, w12) -> (resulting string=→"模块版本号":string)  [unwired: 2 in, 1 out]
  n241 = call "Close TimingControl.vi"("error in (no error)"=w2, "TimingControl in"=w3) -> ()  [unwired: 9 in, 1 out]
